vi "Module Loop.vi"(8 "error in (no error)":errorcluster, 11 "DemoClass in":refnum<class "DemoClass.lvclass">) -> (0 "error out":errorcluster, 3 "DemoClass out":refnum<class "DemoClass.lvclass">)   [LabVIEW 2020, in "VolatusScratch.lvlib" / "DemoClass.lvclass"]
uses:
  DemoClass.lvclass
  C:/dev/lv20CE/relink/lv-volatus/Volatus/Module/Module.lvclass
  Volatus/Module/Module.lvclass/Module.ctl
  Volatus/MessageQ/MessageQ.lvclass/MessageQ.ctl
  Volatus/Module/Module.lvclass
  DemoClass.lvclass/DemoClass.ctl
  Volatus/MessageQ/MessageQ.lvclass
panel:
  in  "Abort":bool
  in  "Start":bool
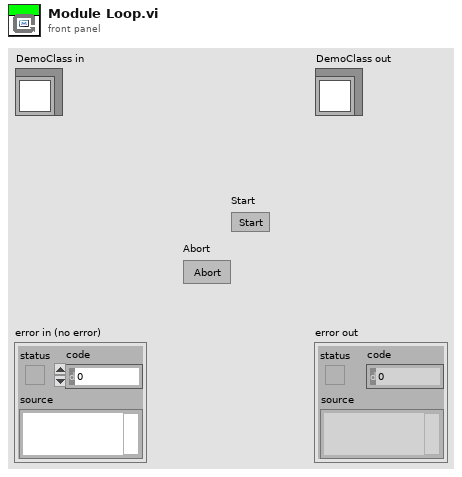
[diagram p1: front panel]
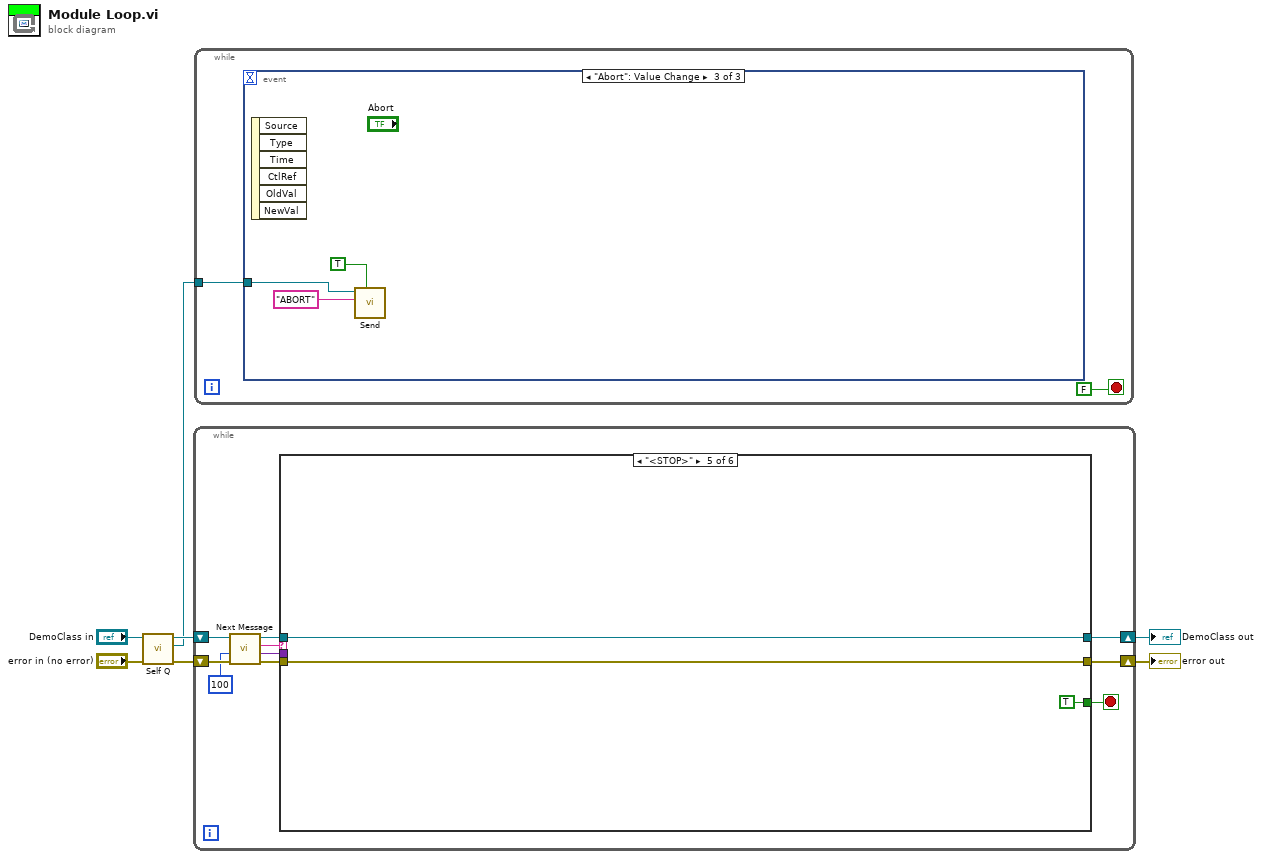
[diagram p0: block diagram]
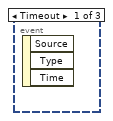
[diagram p2: hidden frame]
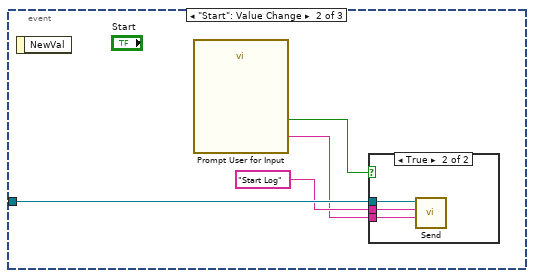
[diagram p3: hidden frame]
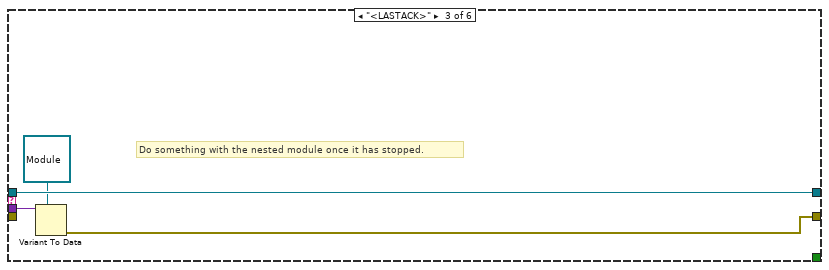
[diagram p7: hidden frame]
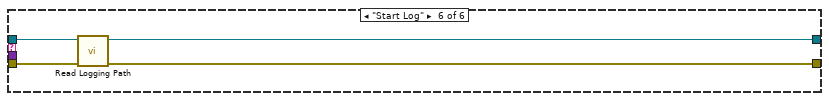
[diagram p9: hidden frame]
diagram:
  n1 = call "Self Q.vi"("Module in"="DemoClass in") -> ("Self Q"=w1:refnum<class "MessageQ.lvclass">, "Module out"=w2:refnum<class "DemoClass.lvclass">)  [unwired: 9 in]
  n2 = while {
    shift-right: [w11] -> w4
    shift-left: w2 -> [w16]
    shift-right: [w10] -> w3
    shift-left: "error in (no error)" -> [w15]
    stop <- w9 stop-if-true
    n3 = call "Next Message.vi"("error in (no error)"=w15, "Timeout ms (-1)"=100, "Module in"=w16) -> ("error out"=w14:errorcluster, "Data"=w8:variant, "ID"=w13:string, "Module out"=w12:refnum<class "DemoClass.lvclass">)  [unwired: 5 in]
    n4 = case shown="\"<STOP>\"" w13 {
      tunnel: w14 -> [w17 w19 _ w25 w28 w33]
      tunnel: w12 -> [w18 w20 w24 w26 w29 w31]
      tunnel: [w18 w20 w24 w26 w29 w30] -> w11
      tunnel: [w17 w19 w21 w25 w28 w32] -> w10
      tunnel: [_ _ _ _ TRUE _] -> w9
      tunnel: w8 -> [_ _ w23 _ _ _]
      frame Default {
      }
      frame "<TIMEOUT>" {
        # "No message for this module was received in time"
      }
      frame "<LASTACK>" {
        # "Do something with the nested module once it has stopped."
        n5 = Variant To Data(type=refnum<class "Module.lvclass"> refnum ("Volatus:Module"), Variant=w23) -> (error out=w21:errorcluster)  [unwired: 1 in, 1 out]
      }
      frame "<CLOSE>" {
      }
      frame "<STOP>" {
      }
      frame "Start Log" {
        n6 = call "Read Logging Path.vi"("error in (no error)"=w33, "DemoClass in"=w31) -> ("error out"=w32:errorcluster, "DemoClass out"=w30:refnum<class "DemoClass.lvclass">)  [unwired: 7 in, 1 out]
      }
    }
  }
  "error out" <- w3
  "DemoClass out" <- w4
  n7 = while {
    tunnel: w1 -> [w35]
    stop <- FALSE stop-if-true
    n8 = event shown="[2] \"Abort\": Value Change" {
      selector: _ -> [_ _ _]
      dyn-events: _ -> [_ _ _]
      timeout: _ -> [_ _ _]
      tunnel: w35 -> [_ w39 w45]
      event Timeout {
        n9 = event-data() -> ()  [unwired: 1 in, 3 out]
      }
      event "Start": Value Change {
        n10 = event-data() -> ()  [unwired: 1 in, 1 out]
        n11 = call "Prompt User for Input"() -> ("Test Name"=w37:string, "OK"=w36:bool)  [unwired: 17 in, 1 out]
        n12 = case shown="True" w36 {
          tunnel: w39 -> [_ w42]
          tunnel: "Start Log" -> [_ w41]
          tunnel: w37 -> [_ w40]
          frame False {
          }
          frame True {
            n13 = call "Send.vi"("Data"=w40, "ID"=w41, "MessageQ in"=w42) -> ()  [unwired: 7 in, 2 out]
          }
        }
      }
      event "Abort": Value Change {
        n14 = event-data() -> ()  [unwired: 1 in, 6 out]
        n15 = call "Send.vi"("High Priority (F)"=TRUE, "ID"="ABORT", "MessageQ in"=w45) -> ()  [unwired: 7 in, 2 out]
      }
    }
  }
